vi "MainClusterToScanParam.vi"(8 "error in (no error)":errorcluster, 9 "Parameters Out":T2={"fastRoundPts"=32, "slowRoundPts"=8, "fastWaveType"=enum."Rounded", "slowWaveType"=enum."Triangle", "fastWavePts"=1024, "slowWavePts"=1024, "outputRateHz"=800000, "yOffset"=0.0, "xOffset"=0.0, "scanSizeSlow"=1e-09, "scanSizeFast"=1e-09, "rotation"=0.0, "timePerLine"=1.0, "numLines"=256, "pointsPerLine"=512, "scanEnable"=FALSE, "slowMoveWavePts"=1024, "slowMoveAccelPts"=128, "moveSpeedSec"=0.2, "singleDirectionScan"=FALSE} {"yOffset" min=0.0 max=1.0 format="%#_6p"; "xOffset" min=0.0 max=1.0 format="%#_6p"; "scanSizeSlow" min=0.0 max=1.0 format="%#_6p"; "scanSizeFast" min=0.0 max=1.0 format="%#_6p"; "timePerLine" min=0.001 max=100.0 format="%#_6ps"; "outputRateHz" format="%.0p"}, 10 "Scan Parameters":T1 {"Scan Rate" format="%.2fHz"; "Lines" format="%#.0f"; "Pixels/Line" format="%#.0f"; "Height" format="%#_6pm"; "Width" format="%#_6pm"; "Time/Line" format="%.2ps"; "Angle" format="%.2f°"; "Y Offset" format="%#_6pm"; "X Offset" format="%#_6pm"}) -> (0 "error out":errorcluster)   [LabVIEW 2016]
uses:
  ScanParametersAllTypeDef.ctl
  controls/ScanWaveform.ctl
  controls/Enum.ctl
panel:
  # "scanWaveFormCtl"
  # "slowMoveParameters"
  # "scanCtl"
  # "ioParams"
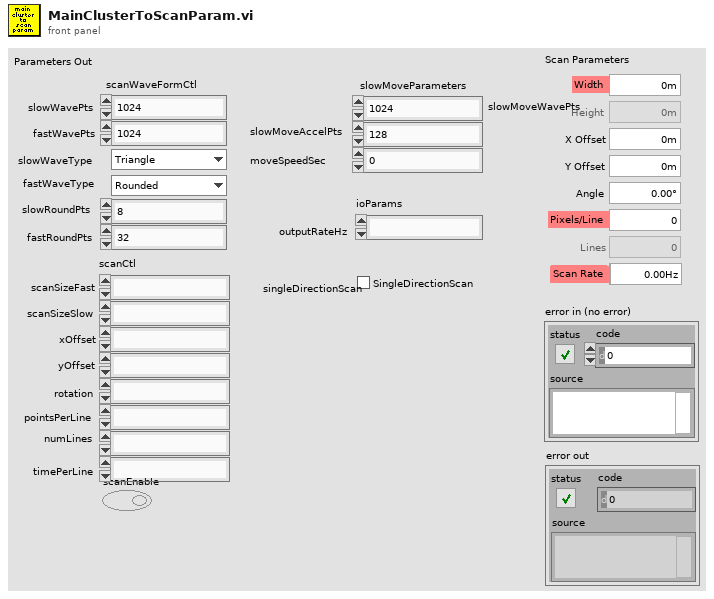
[diagram p1: front panel]
types:
  T1 = cluster{"Width":dbl, "Height":dbl, "X Offset":dbl, "Y Offset":dbl, "Angle":dbl, "Pixels/Line":u32, "Lines":u32, "Time/Line":dbl, "Scan Rate":dbl}
  T2 = typedef "ScanParametersAllTypeDef.ctl" = cluster{"fastRoundPts":u16, "slowRoundPts":u16, "fastWaveType":T3, "slowWaveType":T3, "fastWavePts":u16, "slowWavePts":u16, "outputRateHz":u32, "yOffset":dbl, "xOffset":dbl, "scanSizeSlow":dbl, "scanSizeFast":dbl, "rotation":dbl, "timePerLine":dbl, "numLines":u16, "pointsPerLine":u32, "scanEnable":bool, "slowMoveWavePts":u16, "slowMoveAccelPts":u16, "moveSpeedSec":dbl, "singleDirectionScan":bool}
  T3 = typedef "ScanWaveform.ctl" = enum16{"Sine", "Triangle", "Rounded"}
  T4 = typedef "Enum.ctl" = enum16{"Init", "Read", "Write"}
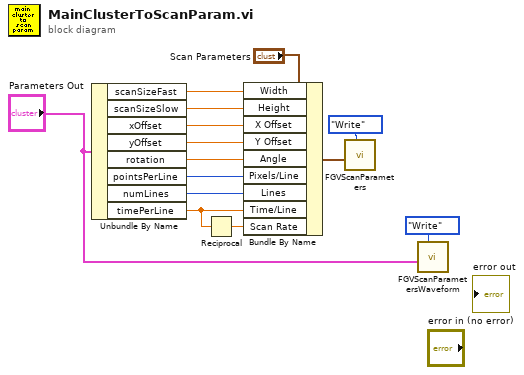
[diagram p0: block diagram]
diagram:
  n1 = Unbundle By Name("Parameters Out") -> ("scanSizeFast"=w6:dbl, "scanSizeSlow"=w7:dbl, "xOffset"=w8:dbl, "yOffset"=w9:dbl, "rotation"=w10:dbl, "pointsPerLine"=w11:u32, "numLines"=w12:u16, "timePerLine"=w5:dbl)
  n2 = Reciprocal(x=w5) -> (1/x=w4:dbl)
  n3 = Bundle By Name(cluster="Scan Parameters", "Width"=w6, "Height"=w7, "X Offset"=w8, "Y Offset"=w9, "Angle"=w10, "Pixels/Line"=w11, "Lines"=w12, "Time/Line"=w5, "Scan Rate"=w4) -> (w13:T1)
  n4 = call "FGVScanParameters.vi"("Enum"=Enum."Write", "Scan Parameters In"=w13) -> ()  [unwired: 8 in, 2 out]
  n5 = call "FGVScanParametersWaveform.vi"("Enum"=Enum."Write", "Parameters In"="Parameters Out") -> ()  [unwired: 8 in, 2 out]
